vi "QuP Multiplexer Control.vi"(11 "Do full quit? (T)":bool=TRUE) -> ()   [LabVIEW 2020, in "QuPMXdriver.lvlib"]
uses:
  QuPMXdriver.lvlib
  91754cce-ab52-4237-b78a-64c01c446f44.vi
  32ad12f4-2c8c-4504-800a-0d774754ae80.vi
  bf4f7028-8ca7-4759-aadb-7144e2be3c91.vi
  040f1b57-66c1-4072-aa26-6ea72dd8171f.vi
  6aed5eb3-691d-4dc6-b830-00691c629857.vi
  3345cd23-f609-4396-914e-6427162a2d46.vi
  Auxiliary/Sequence Editor.vi
  <vilib>/Comparison/Equal/Equal Functor/Equal Functor.lvclass
panel:
  in  "Init-reset":bool caption="Reset after connect:"
  in  "Init-idquery":bool=TRUE caption="ID query after connect:"
  out "FPdisAcon":refnum<vi>[](array[refnum])
  in  "Startup delay (ms)":u32=2000
  in  "disconnect":bool
  out "dummy for event \"check channels\"":bool
  in  "Set to sequence line:":i32=2 min=1 step=1
  in  "set sq line":bool
  out "Connected\nboards":bool[](array[boolean])
  in  "Get sq from MX":bool
  in  "Load sq to MX":bool
  in  "no sequences get":bool
  out "Number of sequence lines:":i32 min=0 step=1
  in  "sequence editor":bool
  out "Guards ref array":refnum<vi>[][](array[refnum])
  in  "G5C1":bool
  in  "G5C2":bool
  in  "G6C1":bool
  in  "G6C2":bool
  in  "G4C1":bool
  in  "G4C2":bool
  in  "G3C1":bool
  in  "G3C2":bool
  in  "G2C1":bool
  in  "G2C2":bool
  in  "G1C1":bool
  in  "G1C2":bool
  out "No. of connected slave boards:":u32
  out "Slaves ref array":refnum<vi>[][](array[refnum])
  in  "S5C1":bool
  in  "S5C2":bool
  in  "S6C1":bool
  in  "S6C2":bool
  in  "S4C1":bool
  in  "S4C2":bool
  in  "S3C1":bool
  in  "S3C2":bool
  in  "S2C1":bool
  in  "S2C2":bool
  in  "S1C1":bool
  in  "S1C2":bool
  in  "connect":bool
  in  "Get Status":bool
  out "Ready?":bool=TRUE
  out "Enabled":bool=TRUE
  in  "check channels":bool
  in  "delay get":bool
  in  "delay set":bool
  in  "Enable\nDelay (ms)":dbl=2.0 min=0.8
  in  "timer get":bool
  in  "timer set":bool
  in  "Timer (ms)":i32=1000 min=0 step=1
  in  "Trigger polarity":enum32{"Positive", "Negative"}(radio)
  in  "Trigger source":enum32{"Internal", "External"}(radio)
  out "FPenAcon":refnum<vi>[](array[refnum])
  in  "Operation":enum32{"Remote", "Local"}(radio)=enum."Local"
  out "ID:":string
  in  "reset":bool
  in  "clear":bool
  in  "stop":bool
  in  "start":bool
  in  "resume":bool
  in  "pause":bool
  in  "Close":bool
  out "error":errorcluster
  in  "VISA":refnum<visa-resource-name>
  # "Connect"
  # "Status"
  # "Channels"
  # "Properties"
  # "Slave boards"
  # "1       2      3      4      5      6"
  # "Channel 1"
  # "Channel 2"
  # "1       2      3      4      5      6"
  # "Guards"
  # "Channel 1"
  # "These are buttons,\nclick it!"
  # "Channel 2"
  # "Sequence"
  # "Error"
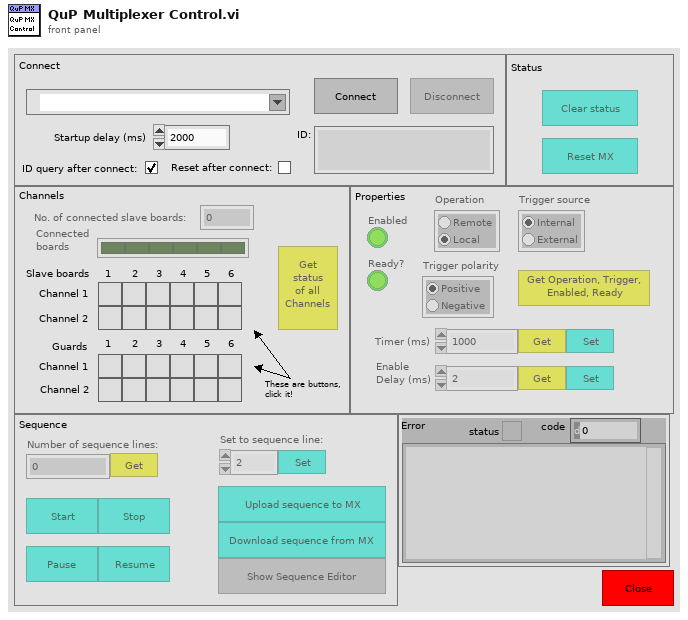
[diagram p1: front panel]
types:
  T1 = enum8{"Enabled", "Disabled", "Disabled and Grayed Out"}
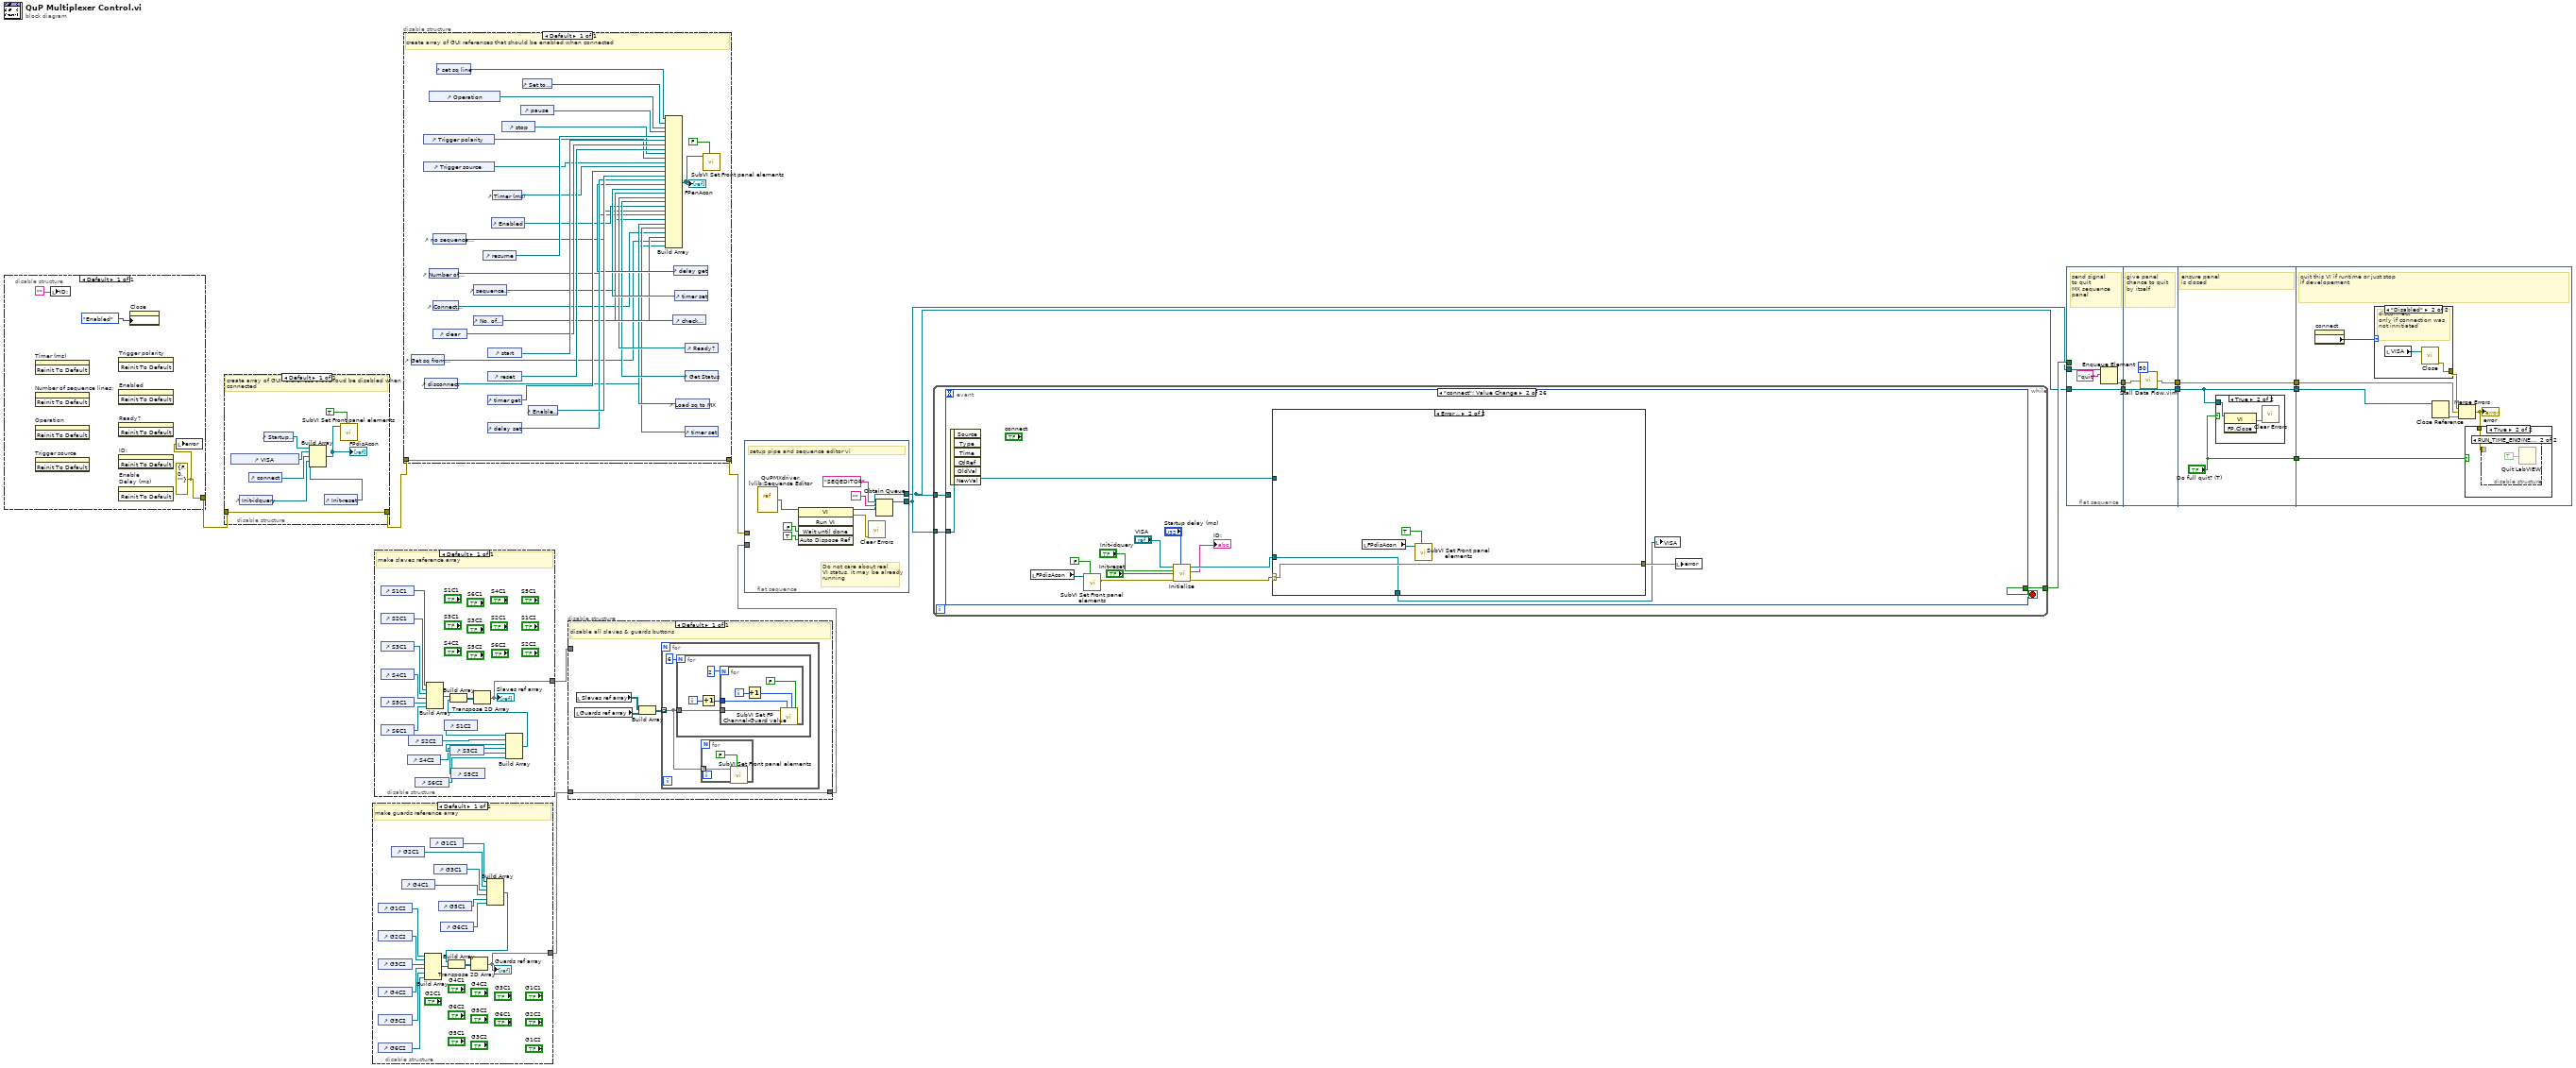
[diagram p0: block diagram]
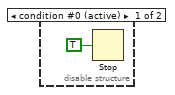
[diagram p4: hidden frame]
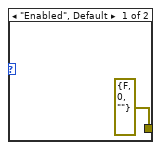
[diagram p5: hidden frame]
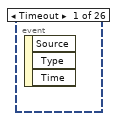
[diagram p6: hidden frame]
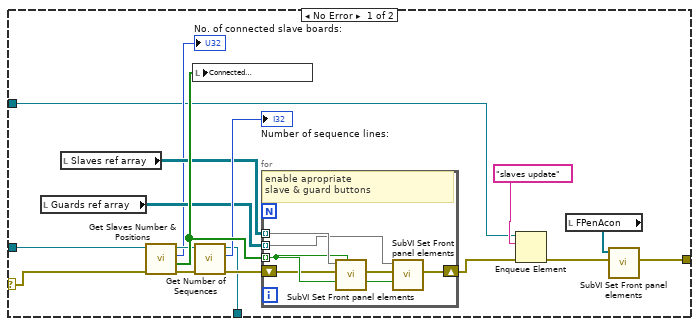
[diagram p7: hidden frame]
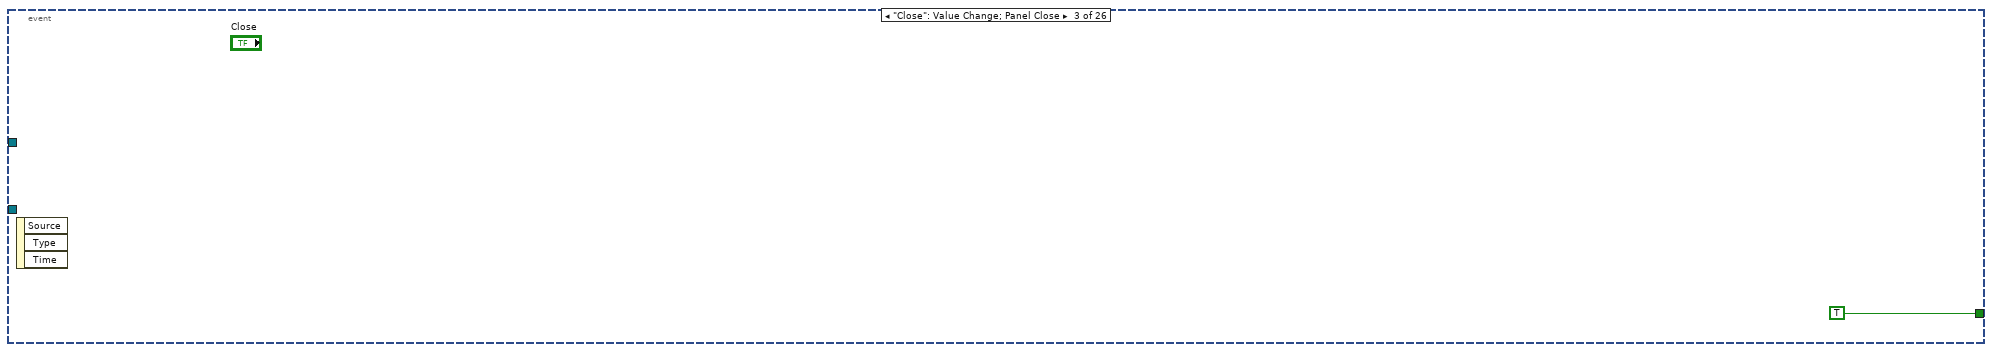
[diagram p8: hidden frame]
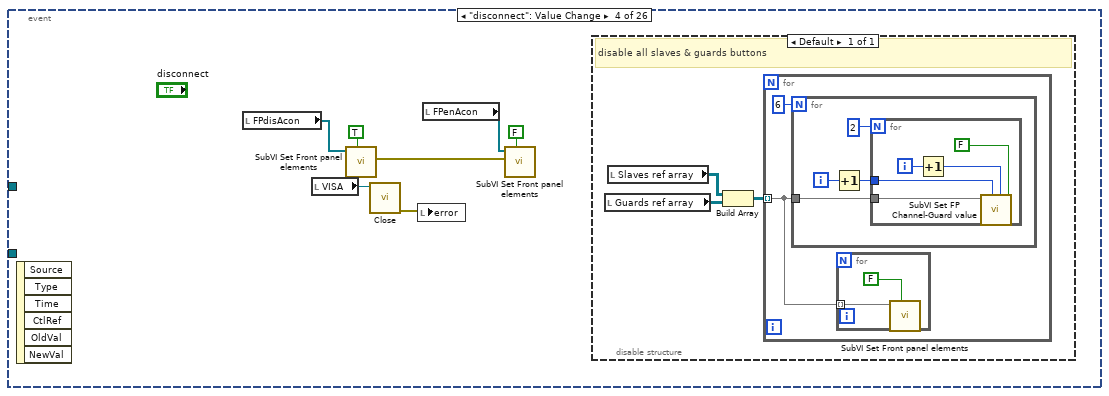
[diagram p9: hidden frame]
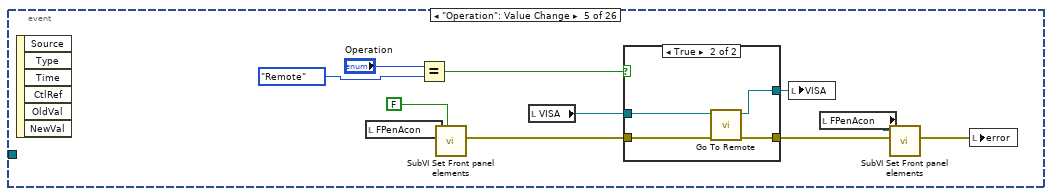
[diagram p10: hidden frame]
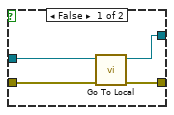
[diagram p11: hidden frame]
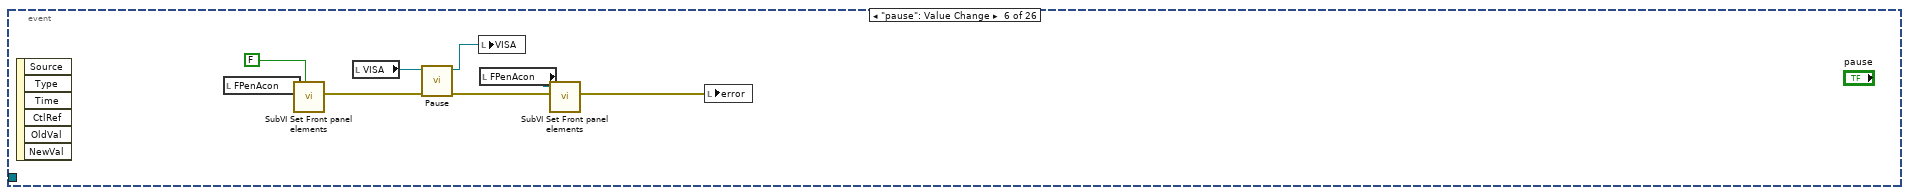
[diagram p12: hidden frame]
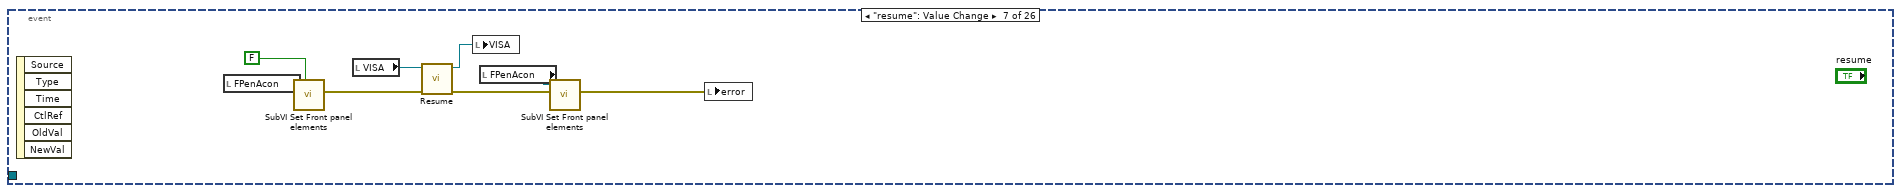
[diagram p13: hidden frame]
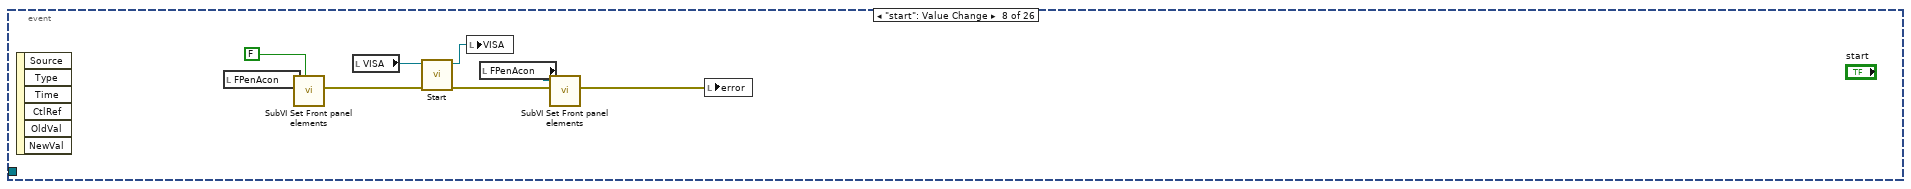
[diagram p14: hidden frame]
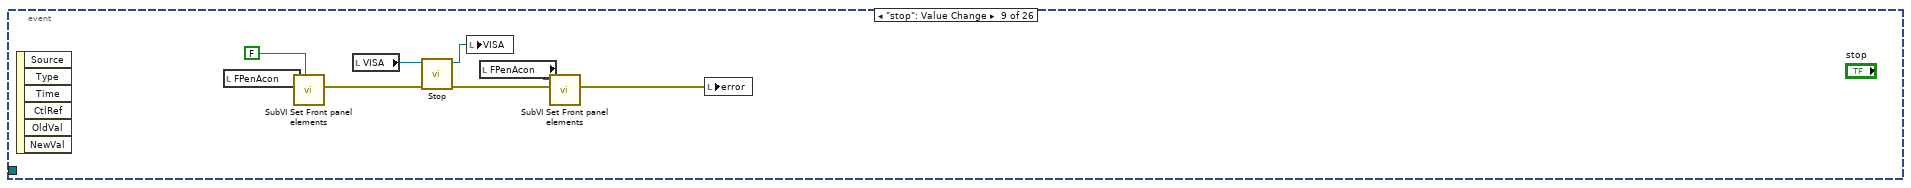
[diagram p15: hidden frame]
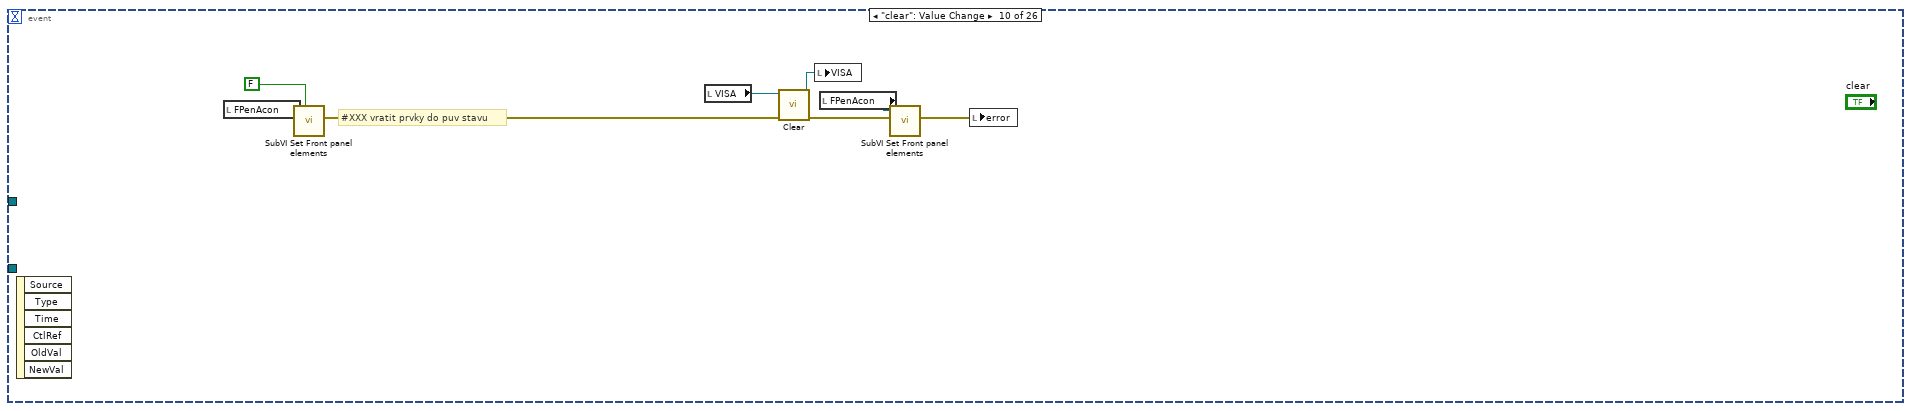
[diagram p16: hidden frame]
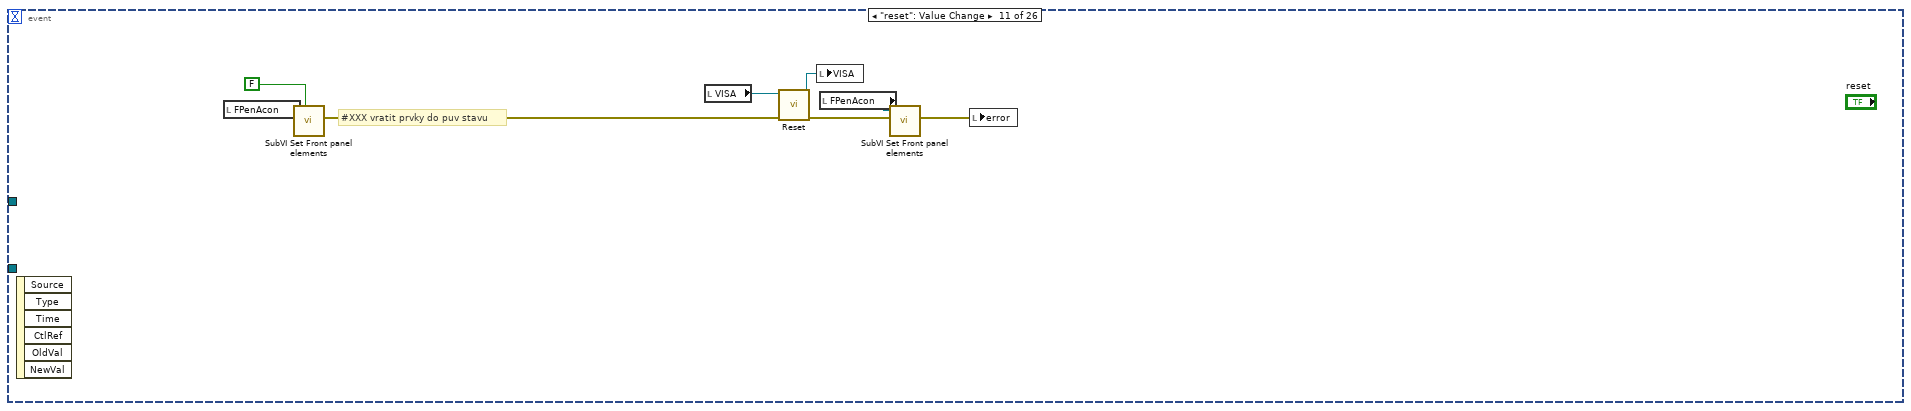
[diagram p17: hidden frame]
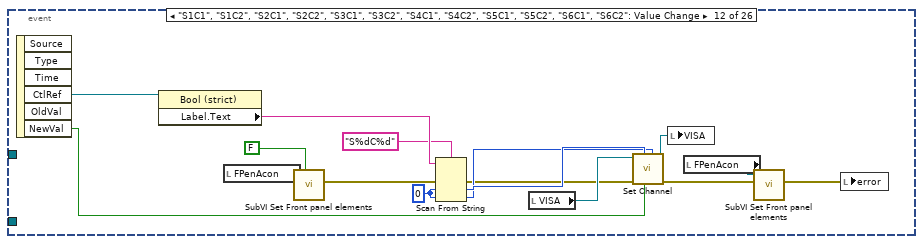
[diagram p18: hidden frame]
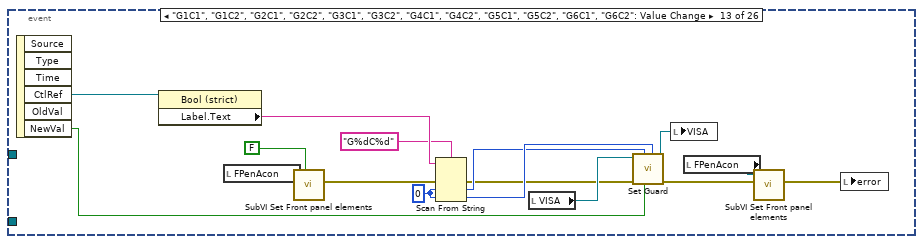
[diagram p19: hidden frame]
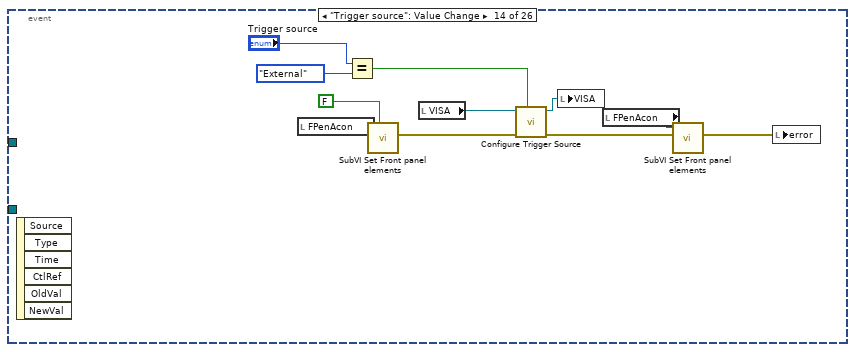
[diagram p20: hidden frame]
diagram:
  n1 = disable-structure shown="Default" {
    disable-tunnel: [w17] -> w6
    frame Enabled {
      w17 = errorcluster {"status"=FALSE, "code"=0, "source"=""} ("error in (no error)")
      n2 = invoke on="Timer (ms)" class="DigNum (strict)" method="Reinit To Default"() -> ()  [unwired: 3 in, 3 out]
      n3 = invoke on="Number of sequence lines:" class="DigNum (strict)" method="Reinit To Default"() -> ()  [unwired: 3 in, 3 out]
      n4 = invoke on="Operation" class="RadioBtnsControl (strict)" method="Reinit To Default"() -> ()  [unwired: 3 in, 3 out]
      n5 = invoke on="Trigger source" class="RadioBtnsControl (strict)" method="Reinit To Default"() -> ()  [unwired: 3 in, 3 out]
      n6 = local write "ID:"("") -> ()
      n7 = invoke on="Trigger polarity" class="RadioBtnsControl (strict)" method="Reinit To Default"() -> ()  [unwired: 3 in, 3 out]
      n8 = invoke on="Enabled" class="Bool (strict)" method="Reinit To Default"() -> ()  [unwired: 3 in, 3 out]
      n9 = invoke on="Ready?" class="Bool (strict)" method="Reinit To Default"() -> ()  [unwired: 3 in, 3 out]
      n10 = invoke on="ID:" class="Str" method="Reinit To Default"() -> ()  [unwired: 3 in, 3 out]
      n11 = invoke on="Enable\nDelay (ms)" class="DigNum (strict)" method="Reinit To Default"() -> ()  [unwired: 3 in, 3 out]
      n12 = property on="Close" class="Bool"("DisabledEnum"=T1."Enabled" ("Disabled")) -> ()  [unwired: 2 in, 2 out]
      n13 = local write "error"(w17) -> ()
    }
  }
  n14 = disable-structure shown="Default" {
    disable-tunnel: [w22] -> w7
    disable-tunnel: w6 -> [w22]
    frame Enabled {
      # "create array of GUI references that shoud be disabled when connected"
      n15 = control-ref of="VISA"() -> (w26:refnum<vi>)
      n16 = control-ref of="Init-idquery"() -> (w21:refnum<vi>)
      n17 = control-ref of="connect"() -> (w25:refnum<vi>)
      n18 = control-ref of="Startup delay (ms)"() -> (w27:refnum<vi>)
      n19 = control-ref of="Init-reset"() -> (w20:refnum<vi>)
      n20 = Build Array(w27, w26, w25, w21, w20) -> (w23:refnum<vi>[])
      "FPdisAcon" <- w23
      n21 = call "SubVI Set Front panel elements.vi"("Enable elements (T)"=TRUE ("Enable elements"), "Array"=w23) -> ()  [unwired: 9 in, 1 out]
    }
  }
  n22 = disable-structure shown="Default" {
    disable-tunnel: [w28] -> w14
    frame Enabled {
      # "make guards reference array"
      n23 = control-ref of="G1C2"() -> (w29:refnum<vi>)
      n24 = control-ref of="G2C2"() -> (w30:refnum<vi>)
      n25 = control-ref of="G3C2"() -> (w31:refnum<vi>)
      n26 = control-ref of="G4C2"() -> (w32:refnum<vi>)
      n27 = control-ref of="G5C2"() -> (w33:refnum<vi>)
      n28 = control-ref of="G6C2"() -> (w34:refnum<vi>)
      n29 = control-ref of="G2C1"() -> (w37:refnum<vi>)
      n30 = control-ref of="G4C1"() -> (w39:refnum<vi>)
      n31 = Build Array(w29, w30, w31, w32, w33, w34) -> (w42:refnum<vi>[])
      n32 = control-ref of="G1C1"() -> (w36:refnum<vi>)
      n33 = control-ref of="G3C1"() -> (w38:refnum<vi>)
      n34 = control-ref of="G5C1"() -> (w40:refnum<vi>)
      n35 = control-ref of="G6C1"() -> (w41:refnum<vi>)
      n36 = Build Array(w36, w37, w38, w39, w40, w41) -> (w35:refnum<vi>[])
      n37 = Build Array(w35, w42) -> (w43:refnum<vi>[][])
      n38 = Transpose 2D Array(2D array=w43) -> (transposed array=w28:refnum<vi>[][])
      "Guards ref array" <- w28
    }
  }
  n39 = disable-structure shown="Default" {
    disable-tunnel: [w44] -> w15
    frame Enabled {
      # "make slaves reference array"
      n40 = control-ref of="S1C1"() -> (w59:refnum<vi>)
      n41 = control-ref of="S2C1"() -> (w58:refnum<vi>)
      n42 = control-ref of="S3C1"() -> (w57:refnum<vi>)
      n43 = control-ref of="S4C1"() -> (w56:refnum<vi>)
      n44 = control-ref of="S5C1"() -> (w55:refnum<vi>)
      n45 = control-ref of="S6C1"() -> (w54:refnum<vi>)
      n46 = control-ref of="S4C2"() -> (w50:refnum<vi>)
      n47 = control-ref of="S2C2"() -> (w52:refnum<vi>)
      n48 = control-ref of="S6C2"() -> (w48:refnum<vi>)
      n49 = Build Array(w59, w58, w57, w56, w55, w54) -> (w46:refnum<vi>[])
      n50 = control-ref of="S1C2"() -> (w53:refnum<vi>)
      n51 = control-ref of="S3C2"() -> (w51:refnum<vi>)
      n52 = control-ref of="S5C2"() -> (w49:refnum<vi>)
      n53 = Build Array(w53, w52, w51, w50, w49, w48) -> (w47:refnum<vi>[])
      n54 = Build Array(w46, w47) -> (w45:refnum<vi>[][])
      n55 = Transpose 2D Array(2D array=w45) -> (transposed array=w44:refnum<vi>[][])
      "Slaves ref array" <- w44
    }
  }
  n56 = disable-structure shown="Default" {
    disable-tunnel: [w67] -> w10
    disable-tunnel: w7 -> [w67]
    frame Enabled {
      # "create array of GUI references that should be enabled when connected"
      n57 = control-ref of="Get sq from MX"() -> (w63:refnum<vi>)
      n58 = control-ref of="Trigger polarity"() -> (w83:refnum<vi>)
      n59 = control-ref of="Trigger source"() -> (w82:refnum<vi>)
      n60 = control-ref of="disconnect"() -> (w60:refnum<vi>)
      n61 = control-ref of="Operation"() -> (w92:refnum<vi>)
      n62 = control-ref of="Number of sequence lines:"() -> (w70:refnum<vi>)
      n63 = control-ref of="no sequences get"() -> (w71:refnum<vi>)
      n64 = control-ref of="Connected\nboards"() -> (w65:refnum<vi>)
      n65 = control-ref of="clear"() -> (w88:refnum<vi>)
      n66 = control-ref of="set sq line"() -> (w61:refnum<vi>)
      n67 = control-ref of="sequence editor"() -> (w69:refnum<vi>)
      n68 = control-ref of="No. of connected slave boards:"() -> (w64:refnum<vi>)
      n69 = control-ref of="resume"() -> (w90:refnum<vi>)
      n70 = control-ref of="start"() -> (w89:refnum<vi>)
      n71 = control-ref of="reset"() -> (w87:refnum<vi>)
      n72 = control-ref of="timer get"() -> (w80:refnum<vi>)
      n73 = control-ref of="delay set"() -> (w78:refnum<vi>)
      n74 = control-ref of="Enabled"() -> (w72:refnum<vi>)
      n75 = control-ref of="Timer (ms)"() -> (w81:refnum<vi>)
      n76 = control-ref of="stop"() -> (w84:refnum<vi>)
      n77 = control-ref of="pause"() -> (w91:refnum<vi>)
      n78 = control-ref of="Set to sequence line:"() -> (w62:refnum<vi>)
      n79 = control-ref of="Enable\nDelay (ms)"() -> (w79:refnum<vi>)
      n80 = control-ref of="check channels"() -> (w75:refnum<vi>)
      n81 = control-ref of="delay get"() -> (w77:refnum<vi>)
      n82 = control-ref of="timer set"() -> (w76:refnum<vi>)
      n83 = control-ref of="Load sq to MX"() -> (w68:refnum<vi>)
      n84 = control-ref of="Ready?"() -> (w74:refnum<vi>)
      n85 = control-ref of="Get Status"() -> (w73:refnum<vi>)
      n86 = control-ref of="timer set"() -> (w66:refnum<vi>)
      n87 = Build Array(w61, w62, w92, w91, w90, w89, w88, w87, w84, w83, w82, w81, w80, w79, w78, w77, w76, w75, w74, w73, w72, w71, w70, w69, w68, w66, w65, w64, w63, w60) -> (w86:refnum<vi>[])
      "FPenAcon" <- w86
      n88 = call "SubVI Set Front panel elements.vi"("Enable elements (T)"=FALSE ("Enable elements"), "Array"=w86) -> ()  [unwired: 9 in, 1 out]
    }
  }
  n89 = disable-structure shown="Default" {
    disable-tunnel: w15 -> [_]
    disable-tunnel: w14 -> [w93]
    disable-tunnel: [w93] -> w11
    frame Enabled {
      # "disable all slaves & guards buttons"
      n90 = local read "Guards ref array"() -> (w94:refnum<vi>[][])
      n91 = local read "Slaves ref array"() -> (w96:refnum<vi>[][])
      n92 = Build Array(w96, w94) -> (w95:refnum<vi>[][][])
      n93 = for {
        tunnel: w95 -> [w97] mode=indexing
        n94 = for {
          N: 6 -> [_]
          tunnel: w97 -> [w102]
          i -> [w100]
          n95 = Increment(x=w100) -> (x+1=w99:i32)
          n96 = for {
            N: 2 -> [_]
            tunnel: w102 -> [w107]
            tunnel: w99 -> [w105]
            i -> [w104]
            n97 = Increment(x=w104) -> (x+1=w103:i32)
            n98 = call "SubVI Set FP Channel-Guard value.vi"("Value"=FALSE, "Ch ID"=w103, "Slave ID"=w105, "Slaves ref array"=w107) -> ()  [unwired: 7 in, 1 out]
          }
        }
        n99 = for {
          tunnel: w97 -> [w109] mode=indexing
          n100 = call "SubVI Set Front panel elements.vi"("Enable elements (T)"=FALSE, "Array"=w109) -> ()  [unwired: 9 in, 1 out]
        }
      }
    }
  }
  n101 = flat-sequence {
    tunnel: [w111] -> w13
    tunnel: [w113] -> w12
    tunnel: w11 -> [_]
    tunnel: w10 -> [_]
    frame #0 {
      # "Do not care about real\nVI status, it may be already\nrunning"
      # "setup pipe and sequence editor vi"
      n102 = vi-ref "QuPMXdriver.lvlib:Sequence Editor.vi"() -> (w117:refnum<vi>)
      n103 = invoke class="VI" method="Run VI"(reference=w117, "Wait until done"=FALSE ("Wait Until Done"), "Auto Dispose Ref"=TRUE ("Wait Until Done")) -> (reference out=w113:refnum<vi>, error out=w110:errorcluster)  [unwired: 2 in, 3 out]
      n104 = call <vilib>:"Clear Errors.vi"("error in (no error)"=w110) -> ()  [unwired: 5 in, 2 out]
      n105 = Obtain Queue(name (unnamed)="SEQEDITOR", element data type="") -> (queue out=w111:refnum<queue>)  [unwired: 3 in, 2 out]
    }
  }
  n106 = while {
    tunnel: [w120] -> w16
    tunnel: w13 -> [w119]
    tunnel: w12 -> [w118]
    stop <- w120 stop-if-true
    n107 = event shown="[1] \"connect\": Value Change" {
      selector: _ -> [_ _ _ _ _ _ _ _ _ _ _ _ _ _ _ _ _ _ _ _ _ _ _ _ _ _]
      dyn-events: _ -> [_ _ _ _ _ _ _ _ _ _ _ _ _ _ _ _ _ _ _ _ _ _ _ _ _ _]
      timeout: _ -> [_ _ _ _ _ _ _ _ _ _ _ _ _ _ _ _ _ _ _ _ _ _ _ _ _ _]
      tunnel: [_ _ TRUE ("Stop") _ _ _ _ _ _ _ _ _ _ _ _ _ _ _ _ _ _ _ _ _ _ _] -> w120
      tunnel: w119 -> [_ w130 _ _ _ _ _ _ _ _ _ _ _ _ _ _ _ _ _ w351 _ _ w420 _ _ w500]
      tunnel: w118 -> [_ _ _ _ _ _ _ _ _ _ _ _ _ _ _ _ _ _ _ _ _ _ _ w425 w475 w503]
      event Timeout {
        n108 = event-data() -> ()  [unwired: 1 in, 3 out]
      }
      event "connect": Value Change {
        n109 = event-data() -> ()  [unwired: 1 in, 6 out]
        n110 = local read "FPdisAcon"() -> (w127:refnum<vi>[])
        n111 = call "SubVI Set Front panel elements.vi"("Enable elements (T)"=FALSE, "Array"=w127) -> ("error out"=w125:errorcluster)  [unwired: 9 in]
        n112 = call "Initialize.vi"("Startup delay (0 ms)"="Startup delay (ms)", "error in (no error)"=w125, "Reset (False)"="Init-reset", "ID Query (True)"="Init-idquery", "VISA resource name"="VISA") -> ("error out"=w124:errorcluster, "ID"=→"ID:":string, "VISA resource name out"=w132:refnum<visa-resource-name>)  [unwired: 4 in]
        n113 = case shown="Error .." w124 {
          selector: w124 -> [w135 w160]
          tunnel: w132 -> [w142 w157]
          tunnel: w130 -> [w137 _]
          tunnel: [w136 w160] -> w128
          tunnel: [w134 w157] -> w121
          frame No Error {
            n114 = local read "Guards ref array"() -> (w145:refnum<vi>[][])
            n115 = local read "Slaves ref array"() -> (w144:refnum<vi>[][])
            n116 = call "Get Slaves Number & Positions.vi"("error in (no error)"=w135, "VISA resource name"=w142) -> ("error out"=w146:errorcluster, "Connected Slaves"=w150:bool[], "No. of Slaves"=→"No. of connected slave boards:":u32, "VISA resource name out"=w148:refnum<visa-resource-name>)  [unwired: 6 in]
            n117 = local write "Connected\nboards"(w150) -> ()
            n118 = call "Get Number of Sequences.vi"("error in (no error)"=w146, "VISA resource name"=w148) -> ("error out"=w147:errorcluster, "Number of sequences"=→"Number of sequence lines:":i32, "VISA resource name out"=w134:refnum<visa-resource-name>)  [unwired: 7 in]
            n119 = for {
              tunnel: w144 -> [w156] mode=indexing
              tunnel: w150 -> [w154] mode=indexing
              tunnel: w145 -> [w155] mode=indexing
              shift-right: [w152] -> w138
              shift-left: w147 -> [w151]
              # "enable apropriate\nslave & guard buttons"
              n120 = call "SubVI Set Front panel elements.vi"("Enable elements (T)"=w154, "error in (passthrough)"=w151, "Array"=w156) -> ("error out"=w153:errorcluster)  [unwired: 8 in]
              n121 = call "SubVI Set Front panel elements.vi"("Enable elements (T)"=w154, "error in (passthrough)"=w153, "Array"=w155) -> ("error out"=w152:errorcluster)  [unwired: 8 in]
            }
            n122 = Enqueue Element(queue=w137, element="slaves update", error in (no error)=w138) -> (error out=w141:errorcluster)  [unwired: 1 in, 2 out]
            n123 = local read "FPenAcon"() -> (w140:refnum<vi>[])
            n124 = call "SubVI Set Front panel elements.vi"("error in (passthrough)"=w141, "Array"=w140) -> ("error out"=w136:errorcluster)  [unwired: 9 in]
          }
          frame Error {
            n125 = local read "FPdisAcon"() -> (w158:refnum<vi>[])
            n126 = call "SubVI Set Front panel elements.vi"("Enable elements (T)"=TRUE, "Array"=w158) -> ()  [unwired: 9 in, 1 out]
          }
        }
        n127 = local write "VISA"(w121) -> ()
        n128 = local write "error"(w128) -> ()
      }
      event "Close": Value Change; Panel Close {
        n129 = event-data() -> ()  [unwired: 1 in, 3 out]
      }
      event "disconnect": Value Change {
        n130 = event-data() -> ()  [unwired: 1 in, 6 out]
        n131 = local read "FPdisAcon"() -> (w163:refnum<vi>[])
        n132 = local read "VISA"() -> (w168:refnum<visa-resource-name>)
        n133 = call "SubVI Set Front panel elements.vi"("Enable elements (T)"=TRUE, "Array"=w163) -> ("error out"=w164:errorcluster)  [unwired: 9 in]
        n134 = call "Close.vi"("VISA resource name"=w168) -> ("error out"=w167:errorcluster)  [unwired: 10 in]
        n135 = local write "error"(w167) -> ()
        n136 = local read "FPenAcon"() -> (w166:refnum<vi>[])
        n137 = call "SubVI Set Front panel elements.vi"("Enable elements (T)"=FALSE, "error in (passthrough)"=w164, "Array"=w166) -> ()  [unwired: 8 in, 1 out]
        n138 = disable-structure shown="Default" {
          frame Enabled {
            # "disable all slaves & guards buttons"
            n139 = local read "Guards ref array"() -> (w169:refnum<vi>[][])
            n140 = local read "Slaves ref array"() -> (w171:refnum<vi>[][])
            n141 = Build Array(w171, w169) -> (w170:refnum<vi>[][][])
            n142 = for {
              tunnel: w170 -> [w172] mode=indexing
              n143 = for {
                N: 6 -> [_]
                tunnel: w172 -> [w177]
                i -> [w175]
                n144 = Increment(x=w175) -> (x+1=w174:i32)
                n145 = for {
                  N: 2 -> [_]
                  tunnel: w177 -> [w182]
                  tunnel: w174 -> [w180]
                  i -> [w179]
                  n146 = Increment(x=w179) -> (x+1=w178:i32)
                  n147 = call "SubVI Set FP Channel-Guard value.vi"("Value"=FALSE, "Ch ID"=w178, "Slave ID"=w180, "Slaves ref array"=w182) -> ()  [unwired: 7 in, 1 out]
                }
              }
              n148 = for {
                tunnel: w172 -> [w184] mode=indexing
                n149 = call "SubVI Set Front panel elements.vi"("Enable elements (T)"=FALSE, "Array"=w184) -> ()  [unwired: 9 in, 1 out]
              }
            }
          }
        }
      }
      event "Operation": Value Change {
        n150 = event-data() -> ()  [unwired: 1 in, 6 out]
        n151 = local read "FPenAcon"() -> (w191:refnum<vi>[])
        n152 = Equal?(x="Operation", y=enum32{"Remote", "Local"}."Remote") -> (x = y?=w192:bool)
        n153 = call "SubVI Set Front panel elements.vi"("Enable elements (T)"=FALSE, "Array"=w191) -> ("error out"=w189:errorcluster)  [unwired: 9 in]
        n154 = local read "VISA"() -> (w195:refnum<visa-resource-name>)
        n155 = case shown="True" w192 {
          tunnel: [w199 w203] -> w188
          tunnel: w195 -> [w198 w202]
          tunnel: w189 -> [w197 w201]
          tunnel: [w196 w200] -> w185
          frame False {
            n156 = call "Go To Local.vi"("error in (no error)"=w197, "VISA resource name"=w198) -> ("error out"=w199:errorcluster, "VISA resource name out"=w196:refnum<visa-resource-name>)  [unwired: 8 in]
          }
          frame True {
            n157 = call "Go To Remote.vi"("error in (no error)"=w201, "VISA resource name"=w202) -> ("error out"=w203:errorcluster, "VISA resource name out"=w200:refnum<visa-resource-name>)  [unwired: 8 in]
          }
        }
        n158 = local write "VISA"(w185) -> ()
        n159 = local read "FPenAcon"() -> (w186:refnum<vi>[])
        n160 = call "SubVI Set Front panel elements.vi"("error in (passthrough)"=w188, "Array"=w186) -> ("error out"=w187:errorcluster)  [unwired: 9 in]
        n161 = local write "error"(w187) -> ()
      }
      event "pause": Value Change {
        n162 = event-data() -> ()  [unwired: 1 in, 6 out]
        n163 = local read "FPenAcon"() -> (w210:refnum<vi>[])
        n164 = call "SubVI Set Front panel elements.vi"("Enable elements (T)"=FALSE, "Array"=w210) -> ("error out"=w207:errorcluster)  [unwired: 9 in]
        n165 = local read "VISA"() -> (w211:refnum<visa-resource-name>)
        n166 = call "Pause.vi"("error in (no error)"=w207, "VISA resource name"=w211) -> ("error out"=w206:errorcluster, "VISA resource name out"=w204:refnum<visa-resource-name>)  [unwired: 8 in]
        n167 = local write "VISA"(w204) -> ()
        n168 = local read "FPenAcon"() -> (w208:refnum<vi>[])
        n169 = call "SubVI Set Front panel elements.vi"("error in (passthrough)"=w206, "Array"=w208) -> ("error out"=w205:errorcluster)  [unwired: 9 in]
        n170 = local write "error"(w205) -> ()
      }
      event "resume": Value Change {
        n171 = event-data() -> ()  [unwired: 1 in, 6 out]
        n172 = local read "FPenAcon"() -> (w217:refnum<vi>[])
        n173 = call "SubVI Set Front panel elements.vi"("Enable elements (T)"=FALSE, "Array"=w217) -> ("error out"=w215:errorcluster)  [unwired: 9 in]
        n174 = local read "VISA"() -> (w219:refnum<visa-resource-name>)
        n175 = call "Resume.vi"("error in (no error)"=w215, "VISA resource name"=w219) -> ("error out"=w214:errorcluster, "VISA resource name out"=w212:refnum<visa-resource-name>)  [unwired: 8 in]
        n176 = local write "VISA"(w212) -> ()
        n177 = local read "FPenAcon"() -> (w218:refnum<vi>[])
        n178 = call "SubVI Set Front panel elements.vi"("error in (passthrough)"=w214, "Array"=w218) -> ("error out"=w213:errorcluster)  [unwired: 9 in]
        n179 = local write "error"(w213) -> ()
      }
      event "start": Value Change {
        n180 = event-data() -> ()  [unwired: 1 in, 6 out]
        n181 = local read "FPenAcon"() -> (w225:refnum<vi>[])
        n182 = call "SubVI Set Front panel elements.vi"("Enable elements (T)"=FALSE, "Array"=w225) -> ("error out"=w223:errorcluster)  [unwired: 9 in]
        n183 = local read "VISA"() -> (w227:refnum<visa-resource-name>)
        n184 = call "Start.vi"("error in (no error)"=w223, "VISA resource name"=w227) -> ("error out"=w222:errorcluster, "VISA resource name out"=w220:refnum<visa-resource-name>)  [unwired: 8 in]
        n185 = local write "VISA"(w220) -> ()
        n186 = local read "FPenAcon"() -> (w226:refnum<vi>[])
        n187 = call "SubVI Set Front panel elements.vi"("error in (passthrough)"=w222, "Array"=w226) -> ("error out"=w221:errorcluster)  [unwired: 9 in]
        n188 = local write "error"(w221) -> ()
      }
      event "stop": Value Change {
        n189 = event-data() -> ()  [unwired: 1 in, 6 out]
        n190 = local read "FPenAcon"() -> (w233:refnum<vi>[])
        n191 = call "SubVI Set Front panel elements.vi"("Enable elements (T)"=FALSE, "Array"=w233) -> ("error out"=w231:errorcluster)  [unwired: 9 in]
        n192 = local read "VISA"() -> (w235:refnum<visa-resource-name>)
        n193 = call "Stop.vi"("error in (no error)"=w231, "VISA resource name"=w235) -> ("error out"=w230:errorcluster, "VISA resource name out"=w228:refnum<visa-resource-name>)  [unwired: 8 in]
        n194 = local write "VISA"(w228) -> ()
        n195 = local read "FPenAcon"() -> (w234:refnum<vi>[])
        n196 = call "SubVI Set Front panel elements.vi"("error in (passthrough)"=w230, "Array"=w234) -> ("error out"=w229:errorcluster)  [unwired: 9 in]
        n197 = local write "error"(w229) -> ()
      }
      event "clear": Value Change {
        # "#XXX vratit prvky do puv stavu"
        n198 = event-data() -> ()  [unwired: 1 in, 6 out]
        n199 = local read "FPenAcon"() -> (w241:refnum<vi>[])
        n200 = call "SubVI Set Front panel elements.vi"("Enable elements (T)"=FALSE, "Array"=w241) -> ("error out"=w239:errorcluster)  [unwired: 9 in]
        n201 = local read "VISA"() -> (w243:refnum<visa-resource-name>)
        n202 = call "Clear.vi"("error in (no error)"=w239, "VISA resource name"=w243) -> ("error out"=w238:errorcluster, "VISA resource name out"=w236:refnum<visa-resource-name>)  [unwired: 8 in]
        n203 = local write "VISA"(w236) -> ()
        n204 = local read "FPenAcon"() -> (w242:refnum<vi>[])
        n205 = call "SubVI Set Front panel elements.vi"("error in (passthrough)"=w238, "Array"=w242) -> ("error out"=w237:errorcluster)  [unwired: 9 in]
        n206 = local write "error"(w237) -> ()
      }
      event "reset": Value Change {
        # "#XXX vratit prvky do puv stavu"
        n207 = event-data() -> ()  [unwired: 1 in, 6 out]
        n208 = local read "FPenAcon"() -> (w249:refnum<vi>[])
        n209 = call "SubVI Set Front panel elements.vi"("Enable elements (T)"=FALSE, "Array"=w249) -> ("error out"=w247:errorcluster)  [unwired: 9 in]
        n210 = local read "VISA"() -> (w251:refnum<visa-resource-name>)
        n211 = call "Reset.vi"("error in (no error)"=w247, "VISA resource name"=w251) -> ("error out"=w246:errorcluster, "VISA resource name out"=w244:refnum<visa-resource-name>)  [unwired: 8 in]
        n212 = local write "VISA"(w244) -> ()
        n213 = local read "FPenAcon"() -> (w250:refnum<vi>[])
        n214 = call "SubVI Set Front panel elements.vi"("error in (passthrough)"=w246, "Array"=w250) -> ("error out"=w245:errorcluster)  [unwired: 9 in]
        n215 = local write "error"(w245) -> ()
      }
      event "S1C1", "S1C2", "S2C1", "S2C2", "S3C1", "S3C2", "S4C1", "S4C2", "S5C1", "S5C2", "S6C1", "S6C2": Value Change {
        w253 = 0 ("default value 1")
        n216 = event-data() -> ("CtlRef"=w267:refnum<vi>, "NewVal"=w261:bool)  [unwired: 1 in, 4 out]
        n217 = property class="Bool (strict)"(reference=w267) -> ("Label.Text"=w266:string)  [unwired: 1 in, 2 out]
        n218 = local read "FPenAcon"() -> (w256:refnum<vi>[])
        n219 = call "SubVI Set Front panel elements.vi"("Enable elements (T)"=FALSE, "Array"=w256) -> ("error out"=w254:errorcluster)  [unwired: 9 in]
        n220 = Scan From String(format string="S%dC%d", input string=w266, error in=w254, default 1=w253, default 2=w253) -> (error out=w260:errorcluster, output 1=w264:i32, output 2=w263:i32)  [unwired: 1 in, 2 out]
        n221 = local read "VISA"() -> (w262:refnum<visa-resource-name>)
        n222 = call "Set Channel.vi"("Channel"=w263, "Channel Status"=w261, "Slave"=w264, "error in (no error)"=w260, "VISA resource name"=w262) -> ("error out"=w258:errorcluster, "VISA resource name out"=w252:refnum<visa-resource-name>)  [unwired: 5 in]
        n223 = local write "VISA"(w252) -> ()
        n224 = local read "FPenAcon"() -> (w259:refnum<vi>[])
        n225 = call "SubVI Set Front panel elements.vi"("error in (passthrough)"=w258, "Array"=w259) -> ("error out"=w257:errorcluster)  [unwired: 9 in]
        n226 = local write "error"(w257) -> ()
      }
      event "G1C1", "G1C2", "G2C1", "G2C2", "G3C1", "G3C2", "G4C1", "G4C2", "G5C1", "G5C2", "G6C1", "G6C2": Value Change {
        w275 = 0 ("default value 1")
        n227 = event-data() -> ("CtlRef"=w281:refnum<vi>, "NewVal"=w277:bool)  [unwired: 1 in, 4 out]
        n228 = property class="Bool (strict)"(reference=w281) -> ("Label.Text"=w283:string)  [unwired: 1 in, 2 out]
        n229 = local read "FPenAcon"() -> (w274:refnum<vi>[])
        n230 = call "SubVI Set Front panel elements.vi"("Enable elements (T)"=FALSE, "Array"=w274) -> ("error out"=w272:errorcluster)  [unwired: 9 in]
        n231 = Scan From String(format string="G%dC%d", input string=w283, error in=w272, default 1=w275, default 2=w275) -> (error out=w276:errorcluster, output 1=w279:i32, output 2=w280:i32)  [unwired: 1 in, 2 out]
        n232 = local read "VISA"() -> (w278:refnum<visa-resource-name>)
        n233 = call "Set Guard.vi"("Channel"=w280, "Channel Guard Status"=w277, "Slave"=w279, "error in (no error)"=w276, "VISA resource name"=w278) -> ("error out"=w270:errorcluster, "VISA resource name out"=w268:refnum<visa-resource-name>)  [unwired: 5 in]
        n234 = local write "VISA"(w268) -> ()
        n235 = local read "FPenAcon"() -> (w271:refnum<vi>[])
        n236 = call "SubVI Set Front panel elements.vi"("error in (passthrough)"=w270, "Array"=w271) -> ("error out"=w269:errorcluster)  [unwired: 9 in]
        n237 = local write "error"(w269) -> ()
      }
      event "Trigger source": Value Change {
        n238 = event-data() -> ()  [unwired: 1 in, 6 out]
        n239 = local read "FPenAcon"() -> (w292:refnum<vi>[])
        n240 = Equal?(x="Trigger source", y=enum32{"Internal", "External"}."External") -> (x = y?=w286:bool)
        n241 = call "SubVI Set Front panel elements.vi"("Enable elements (T)"=FALSE, "Array"=w292) -> ("error out"=w288:errorcluster)  [unwired: 9 in]
        n242 = local read "VISA"() -> (w290:refnum<visa-resource-name>)
        n243 = call "Configure Trigger Source.vi"("Trigger External (T)"=w286, "error in (no error)"=w288, "VISA resource name"=w290) -> ("error out"=w289:errorcluster, "VISA resource name out"=w284:refnum<visa-resource-name>)  [unwired: 7 in]
        n244 = local write "VISA"(w284) -> ()
        n245 = local read "FPenAcon"() -> (w293:refnum<vi>[])
        n246 = call "SubVI Set Front panel elements.vi"("error in (passthrough)"=w289, "Array"=w293) -> ("error out"=w294:errorcluster)  [unwired: 9 in]
        n247 = local write "error"(w294) -> ()
      }
      event "Trigger polarity": Value Change {
        n248 = event-data() -> ()  [unwired: 1 in, 6 out]
        n249 = local read "FPenAcon"() -> (w303:refnum<vi>[])
        n250 = Equal?(x="Trigger polarity", y=enum32{"Positive", "Negative"}."Positive") -> (x = y?=w297:bool)
        n251 = call "SubVI Set Front panel elements.vi"("Enable elements (T)"=FALSE, "Array"=w303) -> ("error out"=w301:errorcluster)  [unwired: 9 in]
        n252 = local read "VISA"() -> (w296:refnum<visa-resource-name>)
        n253 = call "Configure Trigger Polarity.vi"("Trigger Polarity Positive (T)"=w297, "error in (no error)"=w301, "VISA resource name"=w296) -> ("error out"=w300:errorcluster, "VISA resource name out"=w295:refnum<visa-resource-name>)  [unwired: 7 in]
        n254 = local write "VISA"(w295) -> ()
        n255 = local read "FPenAcon"() -> (w304:refnum<vi>[])
        n256 = call "SubVI Set Front panel elements.vi"("error in (passthrough)"=w300, "Array"=w304) -> ("error out"=w305:errorcluster)  [unwired: 9 in]
        n257 = local write "error"(w305) -> ()
      }
      event "timer set": Value Change {
        n258 = event-data() -> ()  [unwired: 1 in, 6 out]
        n259 = To Double Precision Float(number="Timer (ms)") -> (double precision float=w311:dbl)
        n260 = local read "FPenAcon"() -> (w314:refnum<vi>[])
        n261 = expression code="x/1000"(w311) -> (w310:dbl)
        n262 = call "SubVI Set Front panel elements.vi"("Enable elements (T)"=FALSE, "Array"=w314) -> ("error out"=w308:errorcluster)  [unwired: 9 in]
        n263 = local read "VISA"() -> (w309:refnum<visa-resource-name>)
        n264 = call "Configure Timer.vi"("error in (no error)"=w308, "Internal timer (2 s)"=w310, "VISA resource name"=w309) -> ("error out"=w307:errorcluster, "VISA resource name out"=w306:refnum<visa-resource-name>)  [unwired: 7 in]
        n265 = local write "VISA"(w306) -> ()
        n266 = local read "FPenAcon"() -> (w315:refnum<vi>[])
        n267 = call "SubVI Set Front panel elements.vi"("error in (passthrough)"=w307, "Array"=w315) -> ("error out"=w316:errorcluster)  [unwired: 9 in]
        n268 = local write "error"(w316) -> ()
      }
      event "timer get": Value Change {
        n269 = event-data() -> ()  [unwired: 1 in, 6 out]
        n270 = local read "FPenAcon"() -> (w324:refnum<vi>[])
        n271 = call "SubVI Set Front panel elements.vi"("Enable elements (T)"=FALSE, "Array"=w324) -> ("error out"=w322:errorcluster)  [unwired: 9 in]
        n272 = local read "VISA"() -> (w320:refnum<visa-resource-name>)
        n273 = call "Get Timer.vi"("error in (no error)"=w322, "VISA resource name"=w320) -> ("error out"=w321:errorcluster, "Internal Timer value (s)"=w319:dbl, "VISA resource name out"=w317:refnum<visa-resource-name>)  [unwired: 7 in]
        n274 = local write "VISA"(w317) -> ()
        n275 = local read "FPenAcon"() -> (w325:refnum<vi>[])
        n276 = expression code="int(x*1000)"(w319) -> (w318:dbl)
        n277 = call "SubVI Set Front panel elements.vi"("error in (passthrough)"=w321, "Array"=w325) -> ("error out"=w326:errorcluster)  [unwired: 9 in]
        n278 = local write "Timer (ms)"(w318) -> ()
        n279 = local write "error"(w326) -> ()
      }
      event "delay set": Value Change {
        n280 = event-data() -> ()  [unwired: 1 in, 6 out]
        n281 = local read "FPenAcon"() -> (w334:refnum<vi>[])
        n282 = expression code="x/1000"("Enable\nDelay (ms)") -> (w329:dbl)
        n283 = call "SubVI Set Front panel elements.vi"("Enable elements (T)"=FALSE, "Array"=w334) -> ("error out"=w331:errorcluster)  [unwired: 9 in]
        n284 = local read "VISA"() -> (w332:refnum<visa-resource-name>)
        n285 = call "Configure Delay.vi"("error in (no error)"=w331, "Delay (s)"=w329, "VISA resource name"=w332) -> ("error out"=w330:errorcluster, "VISA resource name out"=w327:refnum<visa-resource-name>)  [unwired: 7 in]
        n286 = local write "VISA"(w327) -> ()
        n287 = local read "FPenAcon"() -> (w335:refnum<vi>[])
        n288 = call "SubVI Set Front panel elements.vi"("error in (passthrough)"=w330, "Array"=w335) -> ("error out"=w336:errorcluster)  [unwired: 9 in]
        n289 = local write "error"(w336) -> ()
      }
      event "delay get": Value Change {
        n290 = event-data() -> ()  [unwired: 1 in, 6 out]
        n291 = local read "FPenAcon"() -> (w344:refnum<vi>[])
        n292 = call "SubVI Set Front panel elements.vi"("Enable elements (T)"=FALSE, "Array"=w344) -> ("error out"=w342:errorcluster)  [unwired: 9 in]
        n293 = local read "VISA"() -> (w340:refnum<visa-resource-name>)
        n294 = call "Get Delay.vi"("error in (no error)"=w342, "VISA resource name"=w340) -> ("error out"=w341:errorcluster, "Delay (s)"=w339:dbl, "VISA resource name out"=w337:refnum<visa-resource-name>)  [unwired: 7 in]
        n295 = local write "VISA"(w337) -> ()
        n296 = local read "FPenAcon"() -> (w345:refnum<vi>[])
        n297 = expression code="int(x*1000)"(w339) -> (w338:dbl)
        n298 = call "SubVI Set Front panel elements.vi"("error in (passthrough)"=w341, "Array"=w345) -> ("error out"=w346:errorcluster)  [unwired: 9 in]
        n299 = local write "Enable\nDelay (ms)"(w338) -> ()
        n300 = local write "error"(w346) -> ()
      }
      event "check channels", "dummy for event \"check channels\"": Value Change {
        # "this is only to get possibility\nto start this event case\neven if button \"check channels\"\nis latching"
        n301 = event-data() -> ()  [unwired: 1 in, 6 out]
        n302 = local read "FPenAcon"() -> (w363:refnum<vi>[])
        n303 = call "SubVI Set Front panel elements.vi"("Enable elements (T)"=FALSE, "Array"=w363) -> ("error out"=w356:errorcluster)  [unwired: 9 in]
        n304 = local read "VISA"() -> (w357:refnum<visa-resource-name>)
        n305 = local read "Guards ref array"() -> (w353:refnum<vi>[][])
        n306 = local read "Slaves ref array"() -> (w359:refnum<vi>[][])
        n307 = call "Get Slaves Number & Positions.vi"("error in (no error)"=w356, "VISA resource name"=w357) -> ("error out"=w354:errorcluster, "Connected Slaves"=w358:bool[], "No. of Slaves"=w360:u32, "VISA resource name out"=w348:refnum<visa-resource-name>)  [unwired: 6 in]
        "Connected\nboards" <- w358
        n308 = local write "No. of connected slave boards:"(w360) -> ()
        n309 = for {
          tunnel: w359 -> [w371] mode=indexing
          tunnel: w358 -> [w367] mode=indexing
          shift-right: [w368] -> w355
          shift-left: w354 -> [w370]
          tunnel: w353 -> [w366] mode=indexing
          n310 = call "SubVI Set Front panel elements.vi"("Enable elements (T)"=w367, "error in (passthrough)"=w370, "Array"=w371) -> ("error out"=w369:errorcluster)  [unwired: 8 in]
          n311 = call "SubVI Set Front panel elements.vi"("Enable elements (T)"=w367, "error in (passthrough)"=w369, "Array"=w366) -> ("error out"=w368:errorcluster)  [unwired: 8 in]
        }
        n312 = for {
          N: 2 -> [_]
          shift-right: [w377] -> w350
          shift-left: w355 -> [w376]
          shift-right: [w372] -> w347
          shift-left: w348 -> [w373]
          i -> [w375]
          n313 = Increment(x=w375) -> (x+1=w374:i32)
          n314 = for {
            N: 6 -> [_]
            shift-right: [w387] -> w377
            shift-left: w376 -> [w386]
            tunnel: w374 -> [w382]
            shift-right: [w379] -> w372
            shift-left: w373 -> [w380]
            i -> [w385]
            # "#XXX no way how to check guard status?"
            n315 = Increment(x=w385) -> (x+1=w383:i32)
            n316 = call "Get Channel Status.vi"("Channel"=w382, "Slave"=w383, "error in (no error)"=w386, "VISA resource name"=w380) -> ("error out"=w387:errorcluster, "Channel Enabled"=w381:bool, "VISA resource name out"=w379:refnum<visa-resource-name>)  [unwired: 5 in]
            n317 = local read "Slaves ref array"() -> (w384:refnum<vi>[][])
            n318 = call "SubVI Set FP Channel-Guard value.vi"("Value"=w381, "Ch ID"=w382, "Slave ID"=w383, "Slaves ref array"=w384) -> ()  [unwired: 7 in, 1 out]
          }
        }
        n319 = local write "VISA"(w347) -> ()
        n320 = Enqueue Element(queue=w351, element="slaves update", error in (no error)=w350) -> (error out=w349:errorcluster)  [unwired: 1 in, 2 out]
        n321 = local read "FPenAcon"() -> (w364:refnum<vi>[])
        n322 = call "SubVI Set Front panel elements.vi"("error in (passthrough)"=w349, "Array"=w364) -> ("error out"=w365:errorcluster)  [unwired: 9 in]
        n323 = local write "error"(w365) -> ()
      }
      event "Get Status": Value Change {
        n324 = event-data() -> ()  [unwired: 1 in, 6 out]
        n325 = local read "FPenAcon"() -> (w407:refnum<vi>[])
        n326 = call "SubVI Set Front panel elements.vi"("Enable elements (T)"=FALSE, "Array"=w407) -> ("error out"=w402:errorcluster)  [unwired: 9 in]
        n327 = local read "VISA"() -> (w403:refnum<visa-resource-name>)
        n328 = call "Get MX Status.vi"("error in (no error)"=w402, "VISA resource name"=w403) -> ("error out"=w401:errorcluster, "Ready?"=→"Ready?":bool, "Enabled"=→"Enabled":bool, "VISA resource name out"=w388:refnum<visa-resource-name>, "TRG Polarity Positive"=w396:bool, "Local?"=w400:bool, "TRG External"=w392:bool)  [unwired: 3 in]
        n329 = local write "VISA"(w388) -> ()
        n330 = local read "FPenAcon"() -> (w408:refnum<vi>[])
        n331 = Select(t=enum32{"Remote", "Local"}."Local" ("Operation"), s=w400, f=enum32{"Remote", "Local"}."Remote" ("Operation")) -> (s? t:f=w397:enum32{"Remote", "Local"})
        n332 = Select(t=enum32{"Positive", "Negative"}."Positive" ("Trigger polarity"), s=w396, f=enum32{"Positive", "Negative"}."Negative" ("Trigger polarity")) -> (s? t:f=w393:enum32{"Positive", "Negative"})
        n333 = Select(t=enum32{"Internal", "External"}."External" ("Trigger source"), s=w392, f=enum32{"Internal", "External"}."Internal" ("Trigger source")) -> (s? t:f=w389:enum32{"Internal", "External"})
        n334 = call "SubVI Set Front panel elements.vi"("error in (passthrough)"=w401, "Array"=w408) -> ("error out"=w409:errorcluster)  [unwired: 9 in]
        n335 = local write "Operation"(w397) -> ()
        n336 = local write "Trigger polarity"(w393) -> ()
        n337 = local write "Trigger source"(w389) -> ()
        n338 = local write "error"(w409) -> ()
      }
      event "no sequences get": Value Change {
        n339 = event-data() -> ()  [unwired: 1 in, 6 out]
        n340 = local read "FPenAcon"() -> (w416:refnum<vi>[])
        n341 = call "SubVI Set Front panel elements.vi"("Enable elements (T)"=FALSE, "Array"=w416) -> ("error out"=w414:errorcluster)  [unwired: 9 in]
        n342 = local read "VISA"() -> (w412:refnum<visa-resource-name>)
        n343 = call "Get Number of Sequences.vi"("error in (no error)"=w414, "VISA resource name"=w412) -> ("error out"=w413:errorcluster, "Number of sequences"=w411:i32, "VISA resource name out"=w410:refnum<visa-resource-name>)  [unwired: 7 in]
        n344 = local write "VISA"(w410) -> ()
        n345 = local read "FPenAcon"() -> (w417:refnum<vi>[])
        n346 = local write "Number of sequence lines:"(w411) -> ()
        n347 = call "SubVI Set Front panel elements.vi"("error in (passthrough)"=w413, "Array"=w417) -> ("error out"=w418:errorcluster)  [unwired: 9 in]
        n348 = local write "error"(w418) -> ()
      }
      event "sequence editor": Value Change {
        n349 = event-data() -> ()  [unwired: 1 in, 6 out]
        n350 = Enqueue Element(queue=w420, element="FP open") -> ()  [unwired: 2 in, 3 out]
      }
      event "Load sq to MX": Value Change {
        n351 = event-data() -> ()  [unwired: 1 in, 6 out]
        n352 = disable-structure shown="Default" {
          disable-tunnel: w425 -> [w458]
          disable-tunnel: [w443] -> w424
          disable-tunnel: [w442] -> w423
          frame Enabled {
            # "Get actual values from Sequence editor.vi"
            n353 = property class="VI"(reference=w458) -> ("Panel"=w457:refnum<vi>)  [unwired: 1 in, 2 out]
            n354 = property class="Pnl"(reference=w457) -> (reference out=w444:refnum<vi>, "Controls[]"=w445:refnum<vi>[])  [unwired: 1 in, 1 out]
            n355 = Close Reference(reference=w444) -> ()  [unwired: 1 in, 1 out]
            n356 = Close Reference(reference=w445) -> ()  [unwired: 1 in, 1 out]
            n357 = for {
              tunnel: w445 -> [w460] mode=indexing
              tunnel: [w459] -> w447 mode=indexing
              n358 = property class="Ctl"(reference=w460) -> ("Label.Text"=w459:string)  [unwired: 1 in, 2 out]
            }
            n359 = call "Search Unsorted 1D Array.vim"("element"="Sequence" ("Label.Text"), "unsorted 1D array"=w447) -> ("index of element"=w449:i32)  [unwired: 9 in]
            n360 = call "Search Unsorted 1D Array.vim"("element"="Timing\ndelay" ("Label.Text"), "unsorted 1D array"=w447) -> ("index of element"=w455:i32)  [unwired: 9 in]
            n361 = Index Array(array=w445, index=w449) -> (element=w450:refnum<vi>)
            n362 = property class="Ctl"(reference=w450) -> ("Value"=w451:variant)  [unwired: 1 in, 2 out]
            n363 = Index Array(array=w445, index=w455) -> (element=w454:refnum<vi>)
            n364 = property class="Ctl"(reference=w454) -> ("Value"=w453:variant)  [unwired: 1 in, 2 out]
            n365 = Variant To Data(type=u8[] [] ("Ch. bytes 2"), Variant=w453) -> (data=w442:u8[])  [unwired: 1 in, 1 out]
            n366 = Variant To Data(type=bool[][] [], Variant=w451) -> (data=w443:bool[][])  [unwired: 1 in, 1 out]
          }
        }
        n367 = Array Size(array=w423) -> (size(s)=w422:i32)
        n368 = Equal To 0?(x=w422) -> (x = 0?=w421:bool)
        n369 = case shown="False" w421 {
          tunnel: w424 -> [w432 _]
          tunnel: w423 -> [w431 _]
          frame False {
            n370 = local read "FPenAcon"() -> (w436:refnum<vi>[])
            n371 = call "Sequences to Bytes.vi"("Channel states"=w432) -> ("Ch. bytes 2"=w439:u8[], "Ch. bytes 1"=w440:u8[])  [unwired: 9 in]
            n372 = call "SubVI Set Front panel elements.vi"("Enable elements (T)"=FALSE, "Array"=w436) -> ("error out"=w434:errorcluster)  [unwired: 9 in]
            n373 = local read "VISA"() -> (w433:refnum<visa-resource-name>)
            n374 = call "Load Sequences.vi"("Byte 2 Ch."=w439, "Byte 3 Timing Delay"=w431, "Byte 1 Ch."=w440, "error in (no error)"=w434, "VISA resource name"=w433) -> ("error out"=w429:errorcluster, "VISA resource name out"=w427:refnum<visa-resource-name>)  [unwired: 5 in]
            n375 = local read "FPenAcon"() -> (w437:refnum<vi>[])
            n376 = call "Get Number of Sequences.vi"("error in (no error)"=w429, "VISA resource name"=w427) -> ("error out"=w428:errorcluster, "Number of sequences"=w430:i32, "VISA resource name out"=w426:refnum<visa-resource-name>)  [unwired: 7 in]
            n377 = call "SubVI Set Front panel elements.vi"("error in (passthrough)"=w428, "Array"=w437) -> ("error out"=w438:errorcluster)  [unwired: 9 in]
            n378 = local write "VISA"(w426) -> ()
            n379 = local write "error"(w438) -> ()
            n380 = local write "Number of sequence lines:"(w430) -> ()
          }
          frame True {
            n381 = One Button Dialog(message="Sequence matrix is empty.\nUse sequence editor to create\nsequence or load sequence\nfrom file.") -> ()  [unwired: 1 in, 1 out]
          }
        }
      }
      event "set sq line": Value Change {
        n382 = event-data() -> ()  [unwired: 1 in, 6 out]
        n383 = disable-structure shown="Default" {
          disable-tunnel: w475 -> [w486]
          disable-tunnel: [w476] -> w470
          frame Enabled {
            # "Get actual values from Sequence editor.vi"
            n384 = property class="VI"(reference=w486) -> ("Panel"=w485:refnum<vi>)  [unwired: 1 in, 2 out]
            n385 = property class="Pnl"(reference=w485) -> (reference out=w477:refnum<vi>, "Controls[]"=w478:refnum<vi>[])  [unwired: 1 in, 1 out]
            n386 = Close Reference(reference=w477) -> ()  [unwired: 1 in, 1 out]
            n387 = Close Reference(reference=w478) -> ()  [unwired: 1 in, 1 out]
            n388 = for {
              tunnel: w478 -> [w488] mode=indexing
              tunnel: [w487] -> w480 mode=indexing
              n389 = property class="Ctl"(reference=w488) -> ("Label.Text"=w487:string)  [unwired: 1 in, 2 out]
            }
            n390 = call "Search Unsorted 1D Array.vim"("element"="Sequence" ("Label.Text"), "unsorted 1D array"=w480) -> ("index of element"=w482:i32)  [unwired: 9 in]
            n391 = Index Array(array=w478, index=w482) -> (element=w483:refnum<vi>)
            n392 = property class="Ctl"(reference=w483) -> ("Value"=w484:variant)  [unwired: 1 in, 2 out]
            n393 = Variant To Data(type=bool[][] [], Variant=w484) -> (data=w476:bool[][])  [unwired: 1 in, 1 out]
          }
        }
        n394 = local read "FPenAcon"() -> (w473:refnum<vi>[])
        n395 = Decrement(x="Set to sequence line:") -> (x-1=w462:i32)
        n396 = Index Array(array=w470, index (row)=w462) -> (element=w469:bool[])  [unwired: 1 in]
        n397 = call "SubVI Set Front panel elements.vi"("Enable elements (T)"=FALSE, "Array"=w473) -> ("error out"=w471:errorcluster)  [unwired: 9 in]
        n398 = local read "VISA"() -> (w468:refnum<visa-resource-name>)
        n399 = call "Set Sequence Line.vi"("error in (no error)"=w471, "Sequence Line"=w469, "VISA resource name"=w468) -> ("error out"=w467:errorcluster, "VISA resource name out"=w461:refnum<visa-resource-name>)  [unwired: 7 in]
        n400 = local write "VISA"(w461) -> ()
        n401 = local read "FPenAcon"() -> (w474:refnum<vi>[])
        n402 = call "SubVI Set Front panel elements.vi"("error in (passthrough)"=w467, "Array"=w474) -> ("error out"=w466:errorcluster)  [unwired: 9 in]
        n403 = property on="dummy for event \"check channels\"" class="Bool (strict)"(error in=w466, "Val(Sgnl)"=TRUE) -> (error out=w465:errorcluster)  [unwired: 1 in, 1 out]
        n404 = local write "error"(w465) -> ()
      }
      event "Get sq from MX": Value Change {
        n405 = event-data() -> ()  [unwired: 1 in, 6 out]
        n406 = local read "FPenAcon"() -> (w491:refnum<vi>[])
        n407 = call "SubVI Set Front panel elements.vi"("Enable elements (T)"=FALSE, "Array"=w491) -> ("error out"=w509:errorcluster)  [unwired: 9 in]
        n408 = local read "VISA"() -> (w507:refnum<visa-resource-name>)
        n409 = call "Get Sequences.vi"("error in (no error)"=w509, "VISA resource name"=w507) -> ("error out"=w508:errorcluster, "VISA resource name out"=w489:refnum<visa-resource-name>, "Byte 3 Delay"=w501:u8[], "Byte 2 Ch."=w504:u8[], "Byte 1 Ch."=w505:u8[])  [unwired: 5 in]
        n410 = local write "VISA"(w489) -> ()
        n411 = Array Size(array=w501) -> (size(s)=w506:i32)
        n412 = local read "FPenAcon"() -> (w510:refnum<vi>[])
        n413 = call "Bytes to Sequences.vi"("Ch. bytes 2"=w504, "Ch. bytes 1"=w505) -> ("Array"=w502:bool[][])  [unwired: 9 in]
        n414 = call "SubVI Set Front panel elements.vi"("error in (passthrough)"=w508, "Array"=w510) -> ("error out"=w511:errorcluster)  [unwired: 9 in]
        n415 = local write "Number of sequence lines:"(w506) -> ()
        n416 = local write "error"(w511) -> ()
        n417 = disable-structure shown="Default" {
          disable-tunnel: w503 -> [w525]
          disable-tunnel: w502 -> [w514]
          disable-tunnel: w501 -> [w513]
          disable-tunnel: w500 -> [w512]
          disable-tunnel: [w512] -> w492
          frame Enabled {
            # "Push actual values to Sequence editor.vi"
            n418 = property class="VI"(reference=w525) -> ("Panel"=w524:refnum<vi>)  [unwired: 1 in, 2 out]
            n419 = property class="Pnl"(reference=w524) -> (reference out=w515:refnum<vi>, "Controls[]"=w516:refnum<vi>[])  [unwired: 1 in, 1 out]
            n420 = Close Reference(reference=w515) -> ()  [unwired: 1 in, 1 out]
            n421 = Close Reference(reference=w516) -> ()  [unwired: 1 in, 1 out]
            n422 = for {
              tunnel: w516 -> [w527] mode=indexing
              tunnel: [w526] -> w517 mode=indexing
              n423 = property class="Ctl"(reference=w527) -> ("Label.Text"=w526:string)  [unwired: 1 in, 2 out]
            }
            n424 = call "Search Unsorted 1D Array.vim"("element"="Sequence" ("Label.Text"), "unsorted 1D array"=w517) -> ("index of element"=w519:i32)  [unwired: 9 in]
            n425 = call "Search Unsorted 1D Array.vim"("element"="Timing\ndelay" ("Label.Text"), "unsorted 1D array"=w517) -> ("index of element"=w522:i32)  [unwired: 9 in]
            n426 = Index Array(array=w516, index=w519) -> (element=w520:refnum<vi>)
            n427 = property class="Ctl"(reference=w520, "Value"=w514) -> ()  [unwired: 1 in, 2 out]
            n428 = Index Array(array=w516, index=w522) -> (element=w521:refnum<vi>)
            n429 = property class="Ctl"(reference=w521, "Value"=w513) -> ()  [unwired: 1 in, 2 out]
          }
        }
        n430 = Enqueue Element(queue=w492, element="sequence fill missing collumns") -> (queue out=w496:refnum<queue>, error out=w499:errorcluster)  [unwired: 2 in, 1 out]
        n431 = Enqueue Element(queue=w496, element="index timing update", error in (no error)=w499) -> (queue out=w497:refnum<queue>, error out=w498:errorcluster)  [unwired: 1 in, 1 out]
        n432 = Enqueue Element(queue=w497, element="scrollbar sync", error in (no error)=w498) -> ()  [unwired: 1 in, 3 out]
      }
    }
  }
  n433 = flat-sequence {
    tunnel: w12 -> [w531]
    tunnel: w13 -> [w528]
    tunnel: w16 -> [_]
    tunnel: [w531] -> w5
    tunnel: [w529] -> w3
    tunnel: w5 -> [w535]
    tunnel: [w535] -> w4
    tunnel: w3 -> [w534]
    tunnel: [w533] -> w2
    tunnel: [w538] -> w9
    tunnel: w4 -> [w538]
    tunnel: [w537] -> w8
    tunnel: w2 -> [w537]
    tunnel: ["Do full quit? (T)"] -> w1
    tunnel: w9 -> [w545]
    tunnel: w8 -> [w543]
    tunnel: w1 -> [w541]
    frame #0 {
      # "send signal\nto quit\nMX sequence panel"
      n434 = Enqueue Element(queue=w528, element="quit") -> (error out=w529:errorcluster)  [unwired: 2 in, 2 out]
    }
    frame #1 {
      # "give panel \nchance to quit\nby itself"
      n435 = call "Stall Data Flow.vim"("value in"=w534, "milliseconds to wait"=u32 50) -> ("value out"=w533:errorcluster)  [unwired: 1 out]
    }
    frame #2 {
      # "ensure panel\nis closed"
      n436 = case shown="True" "Do full quit? (T)" {
        tunnel: w538 -> [_ w540]
        frame False {
        }
        frame True {
          n437 = invoke class="VI" method="FP.Close"(reference=w540) -> (error out=w539:errorcluster)  [unwired: 2 in, 2 out]
          n438 = call <vilib>:"Clear Errors.vi"("error in (no error)"=w539) -> ()  [unwired: 5 in, 2 out]
        }
      }
    }
    frame #3 {
      # "quit this VI if runtime or just stop\nif developement"
      n439 = property on="connect" class="Bool"() -> ("DisabledEnum"=w542:T1)  [unwired: 2 in, 2 out]
      n440 = case shown="\"Disabled\"" w542 {
        tunnel: [errorcluster {"status"=FALSE, "code"=0, "source"=""} ("error out") w552] -> w547
        frame "Enabled", Default {
        }
        frame "Disabled" {
          # "disconnect\nonly if connection was\nnot innitiated"
          n441 = local read "VISA"() -> (w553:refnum<visa-resource-name>)
          n442 = call "Close.vi"("VISA resource name"=w553) -> ("error out"=w552:errorcluster)  [unwired: 10 in]
        }
      }
      n443 = Close Reference(reference=w545) -> (error out=w544:errorcluster)  [unwired: 1 in]
      n444 = Merge Errors(w547, w543, w544) -> (w546:errorcluster)
      "error" <- w546
      n445 = case shown="True" w541 {
        tunnel: w546 -> [_ w548]
        frame False {
        }
        frame True {
          n446 = disable-structure shown="RUN_TIME_ENGINE==True" {
            disable-tunnel: w548 -> [_ _]
            frame condition #0 (active) {
              n447 = Stop(stop? (T)=TRUE) -> ()
            }
            frame condition #1 {
              n448 = Quit LabVIEW(quit? (T)=TRUE) -> ()
            }
          }
        }
      }
    }
  }
